vi "getConnectionPoints.vi"(0 "reference":refnum<class "AbstractEdge.lvclass">, 5 "error in (no error)":errorcluster) -> (14 "reference out":refnum<class "AbstractEdge.lvclass">, 15 "connectionPoints":T1[](array[typedef]) {"y" format="%.2f"; "x" format="%.2f"}, 19 "error out":errorcluster)   [LabVIEW 2012, in "AbstractEdge.lvclass"]
doc: "public Line2D getConnectionPoints()"
uses:
  <resource>/Framework/Providers/Open_GDS/UML/AbstractEdge_class/AbstractEdge.lvclass
  <resource>/Framework/Providers/Open_GDS/UML/General/Point/Point Point2D.ctl
  <resource>/Framework/Providers/Open_GDS/UML/AbstractNode_class/AbstractNode.lvclass
  <resource>/Framework/Providers/Open_GDS/UML/Direction_class/Direction.lvclass
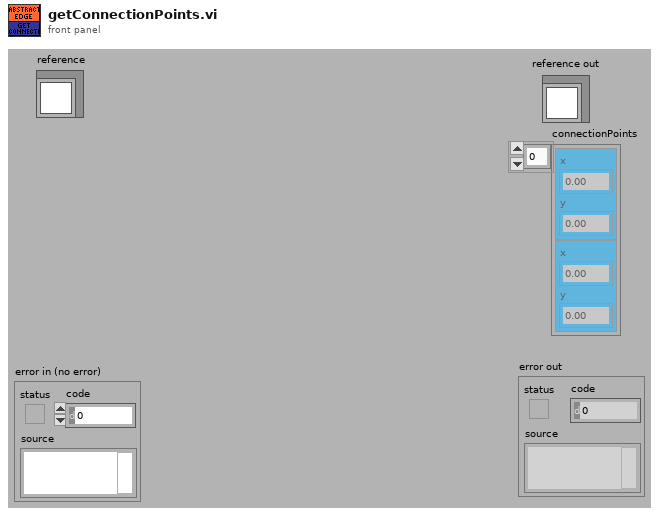
[diagram p1: front panel]
types:
  T1 = typedef "Point Point2D.ctl" = cluster{"x":dbl, "y":dbl}
  T2 = typedef "AbstractEdge.lvclass/ObjectAttributes.ctl" = cluster{"start":refnum<class "AbstractNode.lvclass">, "end":refnum<class "AbstractNode.lvclass">}
  T3 = typedef "Rectangle Rectangle2D.ctl" = cluster{"x":dbl, "y":dbl, "width":dbl, "height":dbl}
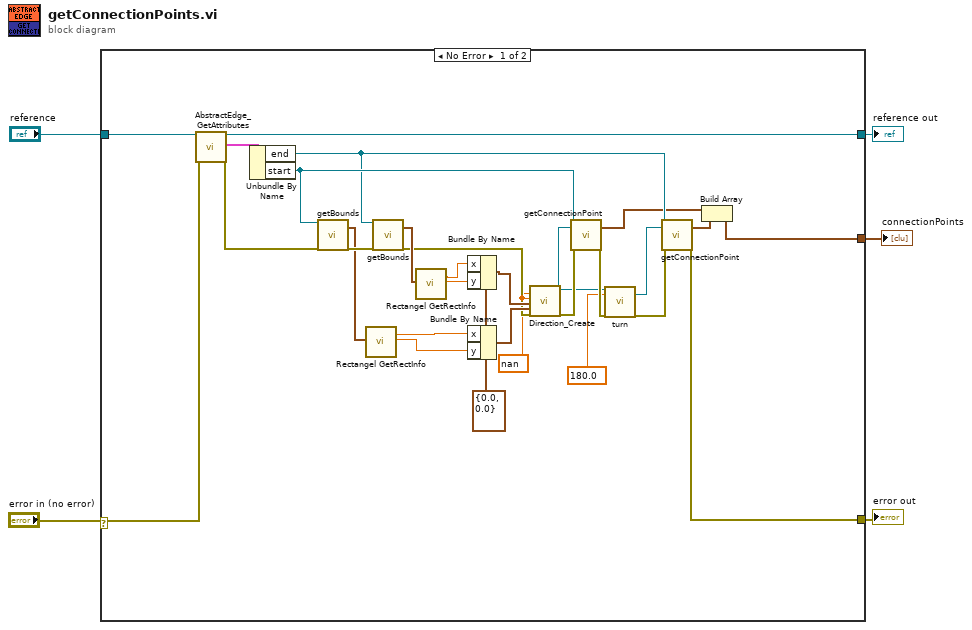
[diagram p0: block diagram]
diagram:
  n1 = case shown="No Error" "error in (no error)" {
    selector: "error in (no error)" -> [w32 w35]
    tunnel: "reference" -> [w34 w36]
    tunnel: [w6 w35] -> w4
    tunnel: [w33 w36] -> w3
    tunnel: [w31 _] -> w1
    frame No Error {
      w22 = T1 {"x"=0.0, "y"=0.0} ("point2D")
      w7 = nan ("dx")
      n2 = call <resource>:"AbstractEdge_GetAttributes.vi"("reference in"=w34, "error in (no error)"=w32) -> ("reference out"=w33:refnum<class "AbstractEdge.lvclass">, "Attributes"=w30:T2, "error out"=w14:errorcluster)  [unwired: 15 out]
      n3 = Unbundle By Name(w30) -> ("end"=w27:refnum<class "AbstractNode.lvclass">, "start"=w28:refnum<class "AbstractNode.lvclass">)
      n4 = call-dynamic "getBounds.vi"("reference"=w28, "error in (no error)"=w14) -> ("bounds"=w26:T3, "error out"=w29:errorcluster)  [unwired: 15 in, 1 out]
      n5 = call <resource>:"Rectangel GetRectInfo.vi"("bounds"=w26) -> ("centerX"=w21:dbl, "centerY"=w20:dbl)  [unwired: 1 in, 16 out]
      n6 = call-dynamic "getBounds.vi"("reference"=w27, "error in (no error)"=w29) -> ("bounds"=w25:T3, "error out"=w17:errorcluster)  [unwired: 15 in, 1 out]
      n7 = call <resource>:"Rectangel GetRectInfo.vi"("bounds"=w25) -> ("centerX"=w23:dbl, "centerY"=w24:dbl)  [unwired: 1 in, 16 out]
      n8 = Bundle By Name(cluster=w22, "x"=w23, "y"=w24) -> (w19:T1)
      n9 = Bundle By Name(cluster=w22, "x"=w21, "y"=w20) -> (w18:T1)
      n10 = call <resource>:"Direction_Create.vi"("dx"=w7, "dy"=w7, "p1"=w19, "p2"=w18, "error in (no error)"=w17) -> ("reference out"=w10:refnum<class "Direction.lvclass">, "error out"=w13:errorcluster)  [unwired: 13 in]
      n11 = call-dynamic "getConnectionPoint.vi"("reference"=w28, "direction"=w10, "error in (no error)"=w13) -> ("point2D"=w16:T1, "error out"=w11:errorcluster)  [unwired: 14 in, 1 out]
      n12 = call <resource>:"turn.vi"("reference"=w10, "angle"=180.0 ("degrees"), "error in (no error)"=w11) -> ("turnedDirection"=w8:refnum<class "Direction.lvclass">, "error out"=w12:errorcluster)  [unwired: 15 out]
      n13 = call-dynamic "getConnectionPoint.vi"("reference"=w27, "direction"=w8, "error in (no error)"=w12) -> ("point2D"=w15:T1, "error out"=w6:errorcluster)  [unwired: 14 in, 1 out]
      n14 = Build Array(w16, w15) -> (w31:T1[])
    }
    frame Error {
    }
  }
  "reference out" <- w3
  "error out" <- w4
  "connectionPoints" <- w1
